vi "Get Size of Data from TD - Digital Waveform (Ramp 256 Samples) - Returns Correct Size.vi"() -> ()   [LabVIEW 2017, in "Composition.Tests.lvlib"]
uses:
  Composition.Tests.lvlib
  <vilib>/Waveform/DWDTOps.llb/Digital Pattern Generator (Ramp).vi
  <vilib>/addons/_JKI Toolkits/Caraya/classes/Assert/Assert Equal Value_Variant.vi
  Composition/Composition.lvlib
  <vilib>/addons/_JKI Toolkits/Caraya/classes/Assert/Assert.lvclass
  <vilib>/addons/_JKI Toolkits/Caraya/classes/Test/Test.lvclass
panel:
  out "error out":errorcluster
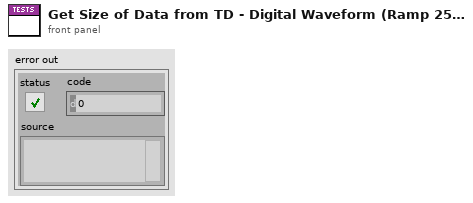
[diagram p1: front panel]
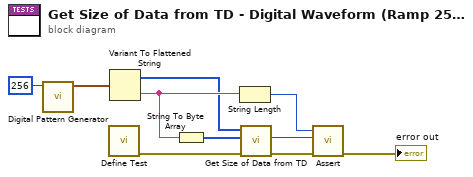
[diagram p0: block diagram]
diagram:
  n1 = call-poly <vilib>:"Digital Pattern Generator.vi"("number of samples"=u32 256) -> ("digital waveform"=w1:digitalwaveform)  [unwired: 9 in, 1 out]
  n2 = call <vilib>:"Define Test.vi"() -> ("error out"=w6:errorcluster)  [unwired: 11 in]
  n3 = Variant To Flattened String(Variant=w1) -> (data string=w9:string, 1:w3:i16[])
  n4 = String To Byte Array(string=w9) -> (unsigned byte array=w4:u8[])
  n5 = String Length(string=w9) -> (length=w7:i32)
  n6 = call "Get Size of Data from TD.vi"("error in (no error)"=w6, "Data String"=w4, "Type Descriptor"=w3) -> ("error out"=w10:errorcluster, "Size of Data"=w5:i32)  [unwired: 7 in]
  n7 = call-poly <vilib>:"Assert.vi"("error in (no error)"=w10, "Y"=w5, "X"=w7) -> ("error out"=→"error out":errorcluster)  [unwired: 8 in]
